vi "MuC_Flush_Buffers.vi"(2 "error in (no error)":errorcluster, 3 "VISA resource name":refnum<visa-resource-name>) -> (0 "error out":errorcluster, 1 "VISA resource name 2":refnum<visa-resource-name>)   [LabVIEW 2018]
doc: "VI to flush the IO buffers of a device.\n\nR. Sheehan 28 - 10 - 2020"
uses:
  <vilib>/Instr/_visa.llb/VISA Flush IO Buffer Mask.ctl
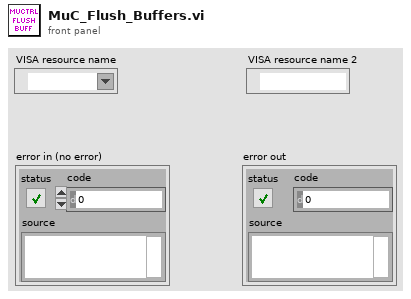
[diagram p1: front panel]
types:
  T1 = typedef "VISA Flush IO Buffer Mask.ctl" = u16
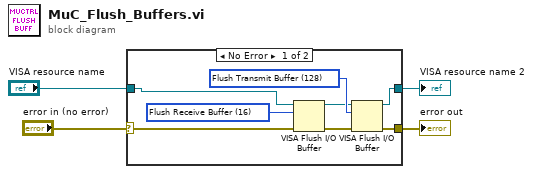
[diagram p0: block diagram]
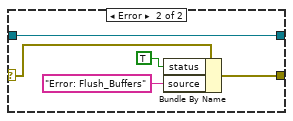
[diagram p2: hidden frame]
diagram:
  n1 = case shown="No Error" "error in (no error)" {
    selector: "error in (no error)" -> [w8 w17]
    tunnel: [w7 w16] -> w3
    tunnel: "VISA resource name" -> [w6 w13]
    tunnel: [w5 w13] -> w1
    frame No Error {
      w9 = T1 16 items=["Flush Receive Buffer"=16, "Write Transmit Buffer to Device"=32, "Flush Receive Buffer (No I/O)"=64, "Flush Transmit Buffer"=128] ("Mask")
      w12 = T1 128 items=["Flush Receive Buffer"=16, "Write Transmit Buffer to Device"=32, "Flush Receive Buffer (No I/O)"=64, "Flush Transmit Buffer"=128] ("Mask")
      n2 = VISA Flush I/O Buffer(VISA resource name=w6, mask (16)=w9, error in (no error)=w8) -> (VISA resource name out=w10:refnum<visa-resource-name>, error out=w11:errorcluster)
      n3 = VISA Flush I/O Buffer(VISA resource name=w10, mask (16)=w12, error in (no error)=w11) -> (VISA resource name out=w5:refnum<visa-resource-name>, error out=w7:errorcluster)
    }
    frame Error {
      n4 = Bundle By Name(cluster=w17, "status"=TRUE, "source"="Error: Flush_Buffers") -> (w16:errorcluster)
    }
  }
  "error out" <- w3
  "VISA resource name 2" <- w1
